vi "Auto Loop 0.vi"(2 "Auto State":u8, 3 "Call Context":T1) -> (0 "Loop 0 Data":T2, 1 "SubState 0":T3=enum."driver control")   [LabVIEW 2013]
uses:
  typedefs/subStates.ctl
  typedefs/Loop Datatypes/Loop 0 Datatype.ctl
  <vilib>/Rock Robotics/WPI/DriverStation/WPI_DriverStationDerivedRobotMode.ctl
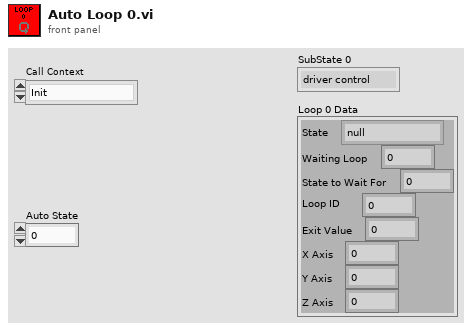
[diagram p1: front panel]
types:
  T1 = typedef "WPI_DriverStationDerivedRobotMode.ctl" = enum16{"Init", "Execute", "Stop"}
  T2 = typedef "Loop 0 Datatype.ctl" = cluster{"State":T3, "Waiting Loop":i32, "State to Wait For":i32, "Loop ID":i32, "Exit Value":i32, "X Axis":dbl, "Y Axis":dbl, "Z Axis":dbl}
  T3 = typedef "subStates.ctl" = enum16{"null", "wait", "driver control", "auto", "manual override", "hold position", "rotate", "feeder", "shoot", "end"}
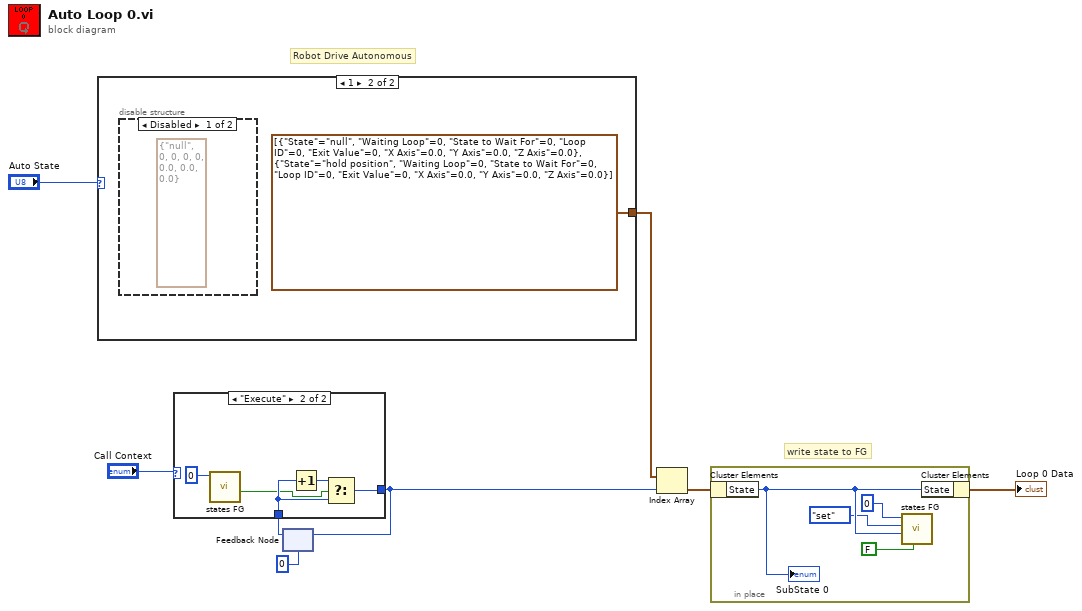
[diagram p0: block diagram]
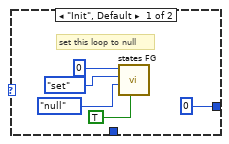
[diagram p2: hidden frame]
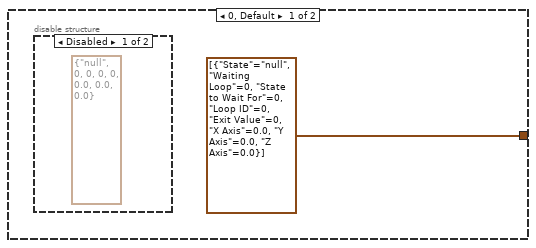
[diagram p3: hidden frame]
diagram:
  # "write state to FG"
  # "Robot Drive Autonomous"
  n1 = case shown="1" "Auto State" {
    tunnel: [T2[] [{"State"=enum."null", "Waiting Loop"=0, "State to Wait For"=0, "Loop ID"=0, "Exit Value"=0, "X Axis"=0.0, "Y Axis"=0.0, "Z Axis"=0.0}] T2[] [{"State"=enum."null", "Waiting Loop"=0, "State to Wait For"=0, "Loop ID"=0, "Exit Value"=0, "X Axis"=0.0, "Y Axis"=0.0, "Z Axis"=0.0}, {"State"=enum."hold position", "Waiting Loop"=0, "State to Wait For"=0, "Loop ID"=0, "Exit Value"=0, "X Axis"=0.0, "Y Axis"=0.0, "Z Axis"=0.0}]] -> w2
    frame 0, Default {
      n2 = disable-structure shown="Disabled" {
        frame Disabled {
          (unwired) T2 {"State"=enum."null", "Waiting Loop"=0, "State to Wait For"=0, "Loop ID"=0, "Exit Value"=0, "X Axis"=0.0, "Y Axis"=0.0, "Z Axis"=0.0} ("Loop 0 Data")
        }
        frame Enabled {
        }
      }
    }
    frame 1 {
      n3 = disable-structure shown="Disabled" {
        frame Disabled {
          (unwired) T2 {"State"=enum."null", "Waiting Loop"=0, "State to Wait For"=0, "Loop ID"=0, "Exit Value"=0, "X Axis"=0.0, "Y Axis"=0.0, "Z Axis"=0.0} ("Loop 0 Data")
        }
        frame Enabled {
        }
      }
    }
  }
  n4 = feedback #1(0) -> (w5:i32)
  n5 = case shown="\"Execute\"" "Call Context" {
    tunnel: w5 -> [_ w19]
    tunnel: [0 w17] -> w1
    frame "Init", Default {
      # "set this loop to null"
      n6 = call "states FG.vi"("exit in"=TRUE, "subState in"=subStates."null", "menu (get)"=enum16{"set", "get"}."set", "Loop ID"=0) -> ()  [unwired: 4 in, 4 out]
    }
    frame "Execute" {
      n7 = call "states FG.vi"("Loop ID"=0) -> ("exit out"=w16:bool)  [unwired: 7 in, 3 out]
      n8 = Increment(x=w19) -> (x+1=w18:i32)
      n9 = Select(t=w18, s=w16, f=w19) -> (s? t:f=w17:i32)
    }
  }
  n10 = feedback-in #1(w1) -> ()
  n11 = Index Array(array=w2, index=w1) -> (element=w4:T2)
  n12 = in-place {
    n13 = in-place-cluster #2(w4) -> ("State"=w22:T3)
    "SubState 0" <- w22
    n14 = call "states FG.vi"("exit in"=FALSE, "subState in"=w22, "menu (get)"=enum16{"set", "get"}."set", "Loop ID"=0) -> ()  [unwired: 4 in, 4 out]
    n15 = in-place-cluster #2("State"=w22) -> (→"Loop 0 Data":T2)
  }
